vi "trace.generate.vi"(10 "trace string":string) -> ()   [LabVIEW 2020, in "Nominal Client.lvclass"]
uses:
  Nominal Client.lvclass
  Nominal Client.lvclass/Nominal Client.ctl
  <vilib>/Utility/SystemLogging/NI_SystemLogging.lvlib
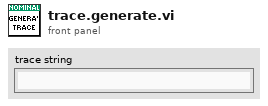
[diagram p1: front panel]
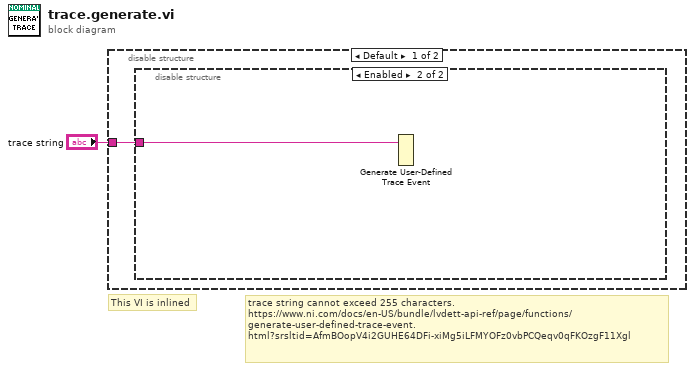
[diagram p0: block diagram]
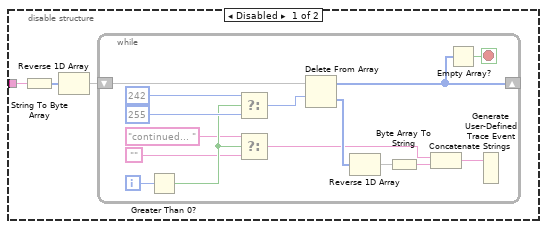
[diagram p2: hidden frame]
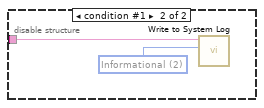
[diagram p3: hidden frame]
diagram:
  # "trace string cannot exceed 255 characters.\nhttps://www.ni.com/docs/en-US/bundle/lvdett-api-ref/page/functions/generate-user-defined-trace-event.html?srsltid=AfmBOopV4i2GUHE64DFi-xiMg5iLFMYOFz0vbPCQeqv0qFKOzgF11Xgl"
  # "This VI is inlined"
  n1 = disable-structure shown="Default" {
    disable-tunnel: "trace string" -> [w2 w23]
    frame condition #0 (active) {
      n2 = disable-structure shown="Enabled" {
        disable-tunnel: w2 -> [w5 w21]
        frame Disabled {
          n3 = String To Byte Array(string=w5) -> (unsigned byte array=w4:u8[])
          n4 = Reverse 1D Array(array=w4) -> (reversed array=w3:u8[])
          n5 = while {
            shift-right: [w17] -> _
            shift-left: w3 -> [w20]
            i -> [w15]
            stop <- w16 stop-if-true
            n6 = Greater Than 0?(x=w15) -> (x > 0?=w9:bool)
            n7 = Select(t=242 ("dimension size"), s=w9, f=255 ("dimension size")) -> (s? t:f=w12:i32)
            n8 = Select(t="continued... " ("trace string"), s=w9, f="") -> (s? t:f=w6:string)
            n9 = Delete From Array(array=w20, length=w12) -> (deleted portion=w19:u8[], array with subset deleted=w17:u8[])  [unwired: 1 in]
            n10 = Reverse 1D Array(array=w19) -> (reversed array=w18:u8[])
            n11 = Byte Array To String(unsigned byte array=w18) -> (string=w11:string)
            n12 = Concatenate Strings(w6, w11) -> (w10:string)
            n13 = Empty Array?(array=w17) -> (empty?=w16:bool)
            n14 = Generate User-Defined Trace Event(2:w10) -> ()  [unwired: 1 in]
          }
        }
        frame Enabled {
          n15 = Generate User-Defined Trace Event(2:w21) -> ()  [unwired: 1 in]
        }
      }
    }
    frame condition #1 {
      w22 = 2 items=["Error", "Warning", "Informational"] ("severity")
      n16 = call <vilib>:"Write to System Log.vi"("severity"=w22, "message"=w23) -> ()  [unwired: 9 in, 1 out]
    }
  }
